vi "getCameraName.vi"(8 "error in (no error)":errorcluster, 11 "WinX32Camera in":refnum<class "WinX32Camera.lvclass">) -> (0 "error out":errorcluster, 2 "Camera":enum16{"Simulation", "Pixis", "ProEM"}(ring), 3 "WinX32Camera out":refnum<class "WinX32Camera.lvclass">)   [LabVIEW 2011, in "WinX32Camera.lvclass"]
uses:
  WinX32Camera.lvclass
  WinX32Camera.lvclass/WinX32Camera.ctl
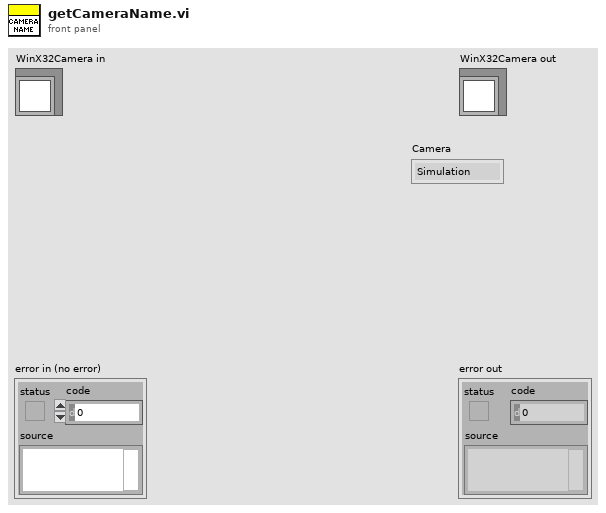
[diagram p1: front panel]
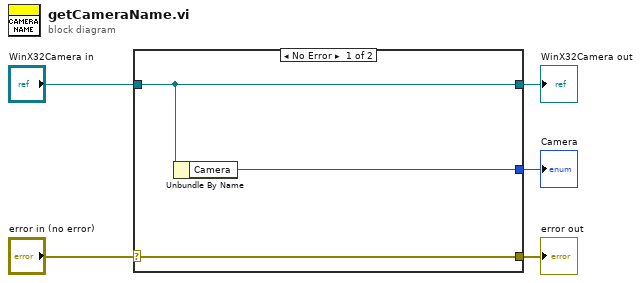
[diagram p0: block diagram]
diagram:
  n1 = case shown="No Error" "error in (no error)" {
    selector: "error in (no error)" -> [w8 w9]
    tunnel: [w8 w9] -> w4
    tunnel: [w7 w10] -> w2
    tunnel: "WinX32Camera in" -> [w7 w10]
    tunnel: [w6 _] -> w1
    frame No Error {
      n2 = Unbundle By Name(w7) -> ("Camera"=w6:enum16{"Simulation", "Pixis", "ProEM"})
    }
    frame Error {
    }
  }
  "error out" <- w4
  "WinX32Camera out" <- w2
  "Camera" <- w1
